vi "addADCScanRateFrame.vi"(8 "error in (no error)":errorcluster, 10 "ModbusBuffer in":refnum<class "ModbusBuffer.lvclass">, 11 "ILC in":refnum<class "ILC.lvclass">) -> (0 "error out":errorcluster, 2 "ModbusBuffer out":refnum<class "ModbusBuffer.lvclass">, 3 "ILC out":refnum<class "ILC.lvclass">)   [LabVIEW 2016, in "RTILC.lvlib" / "ILC.lvclass"]
uses:
  ILC.lvclass
  Common_RT_Modbus/ModbusBuffer/ModbusBuffer.lvclass
  ILC.lvclass/ILC.ctl
  Common_RT_Modbus/DataTypes/ExceptionCodes.ctl
  Common_RT_Modbus/ModbusBuffer/ModbusBuffer.lvclass/ModbusBuffer.ctl
  Common_RT_Modbus/ModbusBuffer/writeByteInstruction.vi
  Common_RT_Modbus/ModbusBuffer/calculateCRC.vi
  Common_RT_Modbus/RTModbus.lvlib
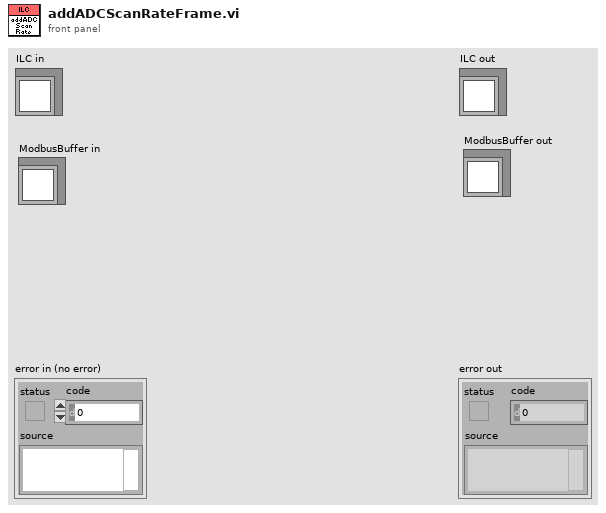
[diagram p1: front panel]
types:
  T1 = typedef "RTModbus.lvlib/ExceptionCodes.ctl" = u16
  T2 = typedef "RTILC.lvlib/ILCScanRates.ctl" = u8
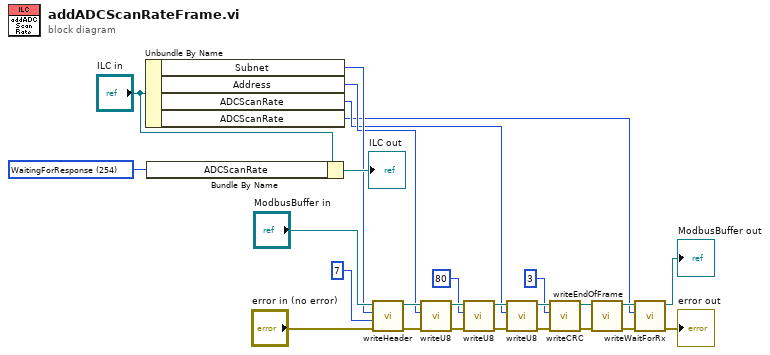
[diagram p0: block diagram]
diagram:
  w26 = T1 254 items=["OK"=0, "IllegalFunction"=1, "IllegalDataAddress"=2, "IllegalDataValue"=3, "SlaveDeviceFailure"=4, "Acknowledge"=5, "SlaveDeviceBusy"=6, "NegativeAcknowledge"=7, "MemoryParityError"=8, "GatewayPathUnavailable"=9, "GatewayTargetDeviceFailedToRespond"=10, "WaitingForResponse"=254, "CRCError"=255] ("ILCData.Responses.ADCOffsetSensitivity")
  n1 = Unbundle By Name("ILC in") -> ("Subnet"=w7:u8, "Address"=w5:u8, "ADCScanRate"=w3:T2, "ADCScanRate"=w1:u32)
  n2 = Bundle By Name(cluster="ILC in", "ADCScanRate"=w26) -> (→"ILC out":refnum<class "ILC.lvclass">)
  n3 = call "writeHeader.vi"("error in (no error)"="error in (no error)", "Length"=u16 7, "Subnet"=w7, "ModbusBuffer in"="ModbusBuffer in") -> ("error out"=w13:errorcluster, "ModbusBuffer out"=w20:refnum<class "ModbusBuffer.lvclass">)  [unwired: 6 in]
  n4 = call "writeU8.vi"("error in (no error)"=w13, "Input"=w5, "ModbusBuffer in"=w20) -> ("error out"=w12:errorcluster, "ModbusBuffer out"=w19:refnum<class "ModbusBuffer.lvclass">)  [unwired: 7 in]
  n5 = call "writeU8.vi"("error in (no error)"=w12, "Input"=u8 80 ("Byte"), "ModbusBuffer in"=w19) -> ("error out"=w23:errorcluster, "ModbusBuffer out"=w22:refnum<class "ModbusBuffer.lvclass">)  [unwired: 7 in]
  n6 = call "writeU8.vi"("error in (no error)"=w23, "Input"=w3, "ModbusBuffer in"=w22) -> ("error out"=w11:errorcluster, "ModbusBuffer out"=w18:refnum<class "ModbusBuffer.lvclass">)  [unwired: 7 in]
  n7 = call "writeCRC.vi"("error in (no error)"=w11, "Length"=3, "ModbusBuffer in"=w18) -> ("error out"=w10:errorcluster, "ModbusBuffer out"=w17:refnum<class "ModbusBuffer.lvclass">)  [unwired: 7 in]
  n8 = call "writeEndOfFrame.vi"("error in (no error)"=w10, "ModbusBuffer in"=w17) -> ("error out"=w9:errorcluster, "ModbusBuffer out"=w16:refnum<class "ModbusBuffer.lvclass">)  [unwired: 8 in]
  n9 = call "writeWaitForRx.vi"("error in (no error)"=w9, "Timeout(us)"=w1, "ModbusBuffer in"=w16) -> ("error out"=→"error out":errorcluster, "ModbusBuffer out"=→"ModbusBuffer out":refnum<class "ModbusBuffer.lvclass">)  [unwired: 7 in]
